vi "SYST_CONF.vi"(0 "VISA IN":refnum<visa-resource-name>, 1 "Address":i32, 5 "error in":errorcluster, 7 "Model":string) -> (14 "VISA Out":refnum<visa-resource-name>, 19 "error out":errorcluster)   [LabVIEW 2018, in "PNA-X.lvlib"]
doc: "SYSTem:CONFigure <model>,<address> \n(Write-only) Restarts as an \"N-port\" PNA using the specified multiport test set. \nLearn more about PNA Multiport capability. \nSee other commands to configure multiport test sets. \nParameters \n<model> String - Model of the test set with which to restart. \nUse \"Native\" to restart without a test set. \nTo see a list of supported test sets, use SENS:MULT:CAT? \n<address> Numeric - GPIB Address of the test set. Ignored when model = \"Native\". \nExamples SYST:CONF \"NATIVE\",0 \nsystem:configure \"N44xx\",18 \nQuery Syntax Not Applicable \nDefault Not Applicable"
uses:
  PNA-X.lvlib
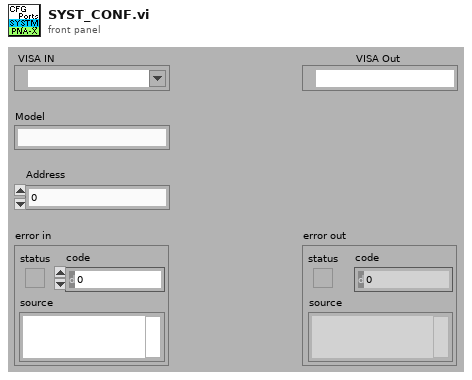
[diagram p1: front panel]
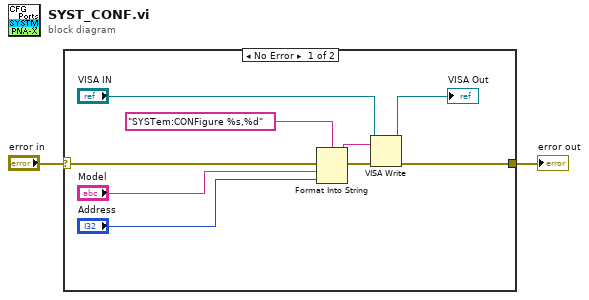
[diagram p0: block diagram]
diagram:
  n1 = case shown="No Error" "error in" {
    selector: "error in" -> [w11 w12]
    tunnel: [w6 w12] -> w1
    frame No Error {
      n2 = Format Into String(format string="SYSTem:CONFigure %s,%d" ("Cmdline"), error in=w11, "Model", "Address") -> (resulting string=w9:string, error out=w10:errorcluster)  [unwired: 1 in]
      n3 = VISA Write(VISA resource name="VISA IN", write buffer=w9, error in (no error)=w10) -> (VISA resource name out=→"VISA Out":refnum<visa-resource-name>, error out=w6:errorcluster)  [unwired: 1 out]
    }
    frame Error {
    }
  }
  "error out" <- w1
